vi "Warn.vi"(8 "NwarnIN":bool, 9 "HwarnIN":bool, 10 "warncontN":T1={"alarmliqN"=90.0, "warn?N"=FALSE, "lessthan?N"=FALSE}, 11 "warncontHe":T2={"alarmliqHe"=85.0, "warn?He"=FALSE, "lessthan?He"=FALSE}) -> (2 "warnNOUT":T1={"alarmliqN"=90.0, "warn?N"=FALSE, "lessthan?N"=FALSE}, 3 "warnHeOUT":T2={"alarmliqHe"=85.0, "warn?He"=FALSE, "lessthan?He"=FALSE})   [LabVIEW 2017, in "Level Meter.lvclass"]
uses:
  Level Meter.lvclass
  Global/Relative Sound Files.vi
panel:
  in  "turnoff":bool
  out "Nwarn":bool caption="LN"
  out "Hwarn":bool caption="LHe"
  in  "exit":bool
  out "disp":string
  out "warn2":bool
  out "warn1":bool
  # "Off"
  # "On"
  # "Greater"
  # "Less"
  # "Off"
  # "On"
  # "Greater"
  # "Less"
  # "Off"
  # "On"
  # "Greater"
  # "Less"
  # "Off"
  # "On"
  # "Greater"
  # "Less"
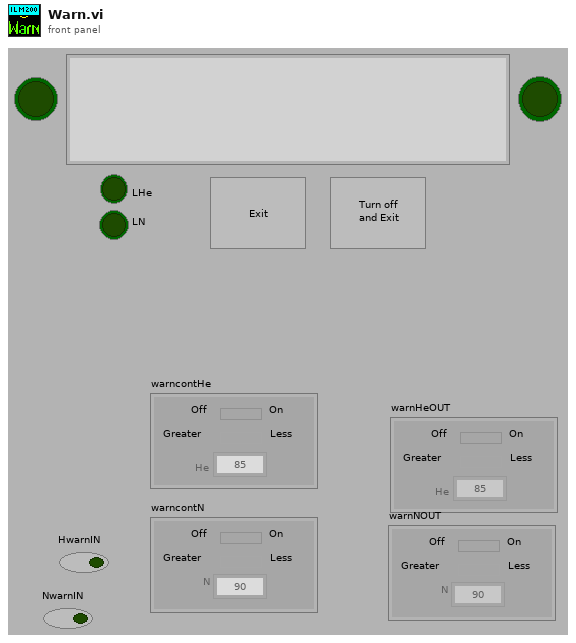
[diagram p1: front panel]
types:
  T1 = cluster{"alarmliqN":dbl, "warn?N":bool, "lessthan?N":bool}
  T2 = cluster{"alarmliqHe":dbl, "warn?He":bool, "lessthan?He":bool}
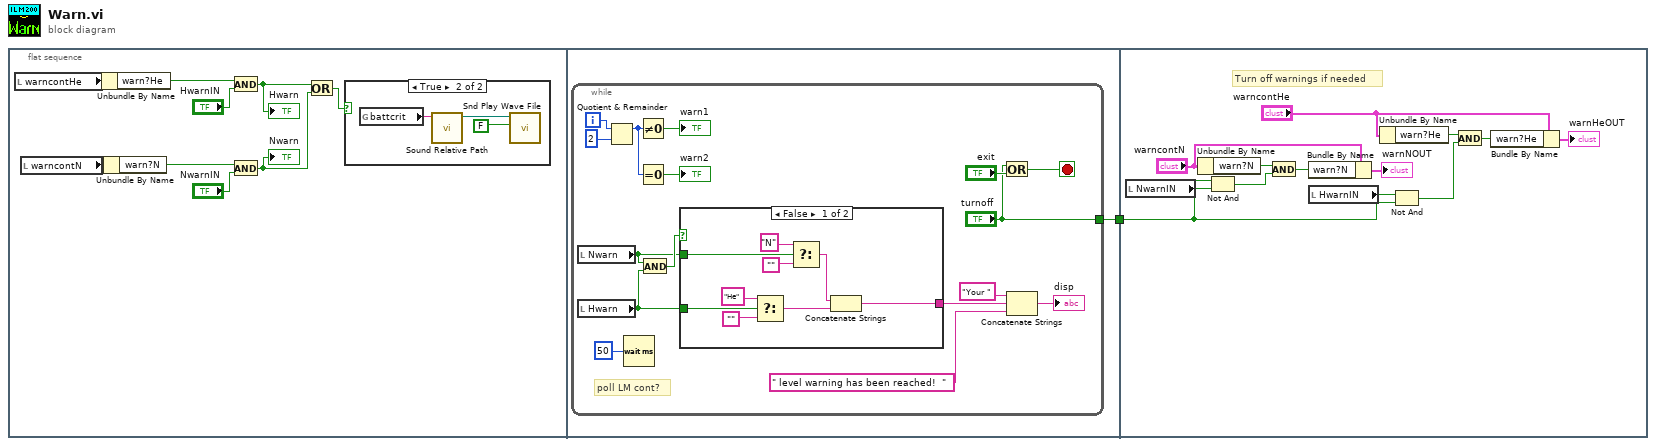
[diagram p0: block diagram]
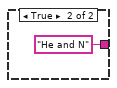
[diagram p3: hidden frame]
diagram:
  n1 = flat-sequence {
    tunnel: [w14] -> w1
    tunnel: w1 -> [w43]
    frame #0 {
      n2 = local read "warncontHe"() -> (w10:T2)
      n3 = local read "warncontN"() -> (w6:T1)
      n4 = Unbundle By Name(w10) -> ("warn?He"=w9:bool)
      n5 = Unbundle By Name(w6) -> ("warn?N"=w7:bool)
      n6 = And(x=w9, y="HwarnIN") -> (x .and. y?=w3:bool)
      "Hwarn" <- w3
      n7 = And(x=w7, y="NwarnIN") -> (x .and. y?=w2:bool)
      "Nwarn" <- w2
      n8 = Or(x=w3, y=w2) -> (x .or. y?=w4:bool)
      n9 = case shown="True" w4 {
        frame False {
        }
        frame True {
          n10 = global read "Relative Sound Files.vi" "battcrit"() -> (w12:string)
          n11 = call "Sound Relative Path.vi"("Sound"=w12) -> ("Relative Path"=w11:path)  [unwired: 10 in]
          n12 = call <vilib>:"Snd Play Wave File.vi"("wait until finish (T)"=FALSE, "wave file path"=w11) -> ()  [unwired: 1 in, 9 out]
        }
      }
    }
    frame #1 {
      n13 = while {
        tunnel: ["turnoff"] -> w14
        i -> [w30]
        stop <- w19 stop-if-true
        # "poll LM cont?"
        n14 = local read "Nwarn"() -> (w26:bool)
        n15 = local read "Hwarn"() -> (w25:bool)
        n16 = Quotient & Remainder(x=w30, y=2) -> (x-y*floor(x/y)=w17:i32)  [unwired: 1 out]
        n17 = Wait (ms)(milliseconds to wait=50) -> ()  [unwired: 1 out]
        n18 = Not Equal To 0?(x=w17) -> (x != 0?=→"warn1":bool)
        n19 = Equal To 0?(x=w17) -> (x = 0?=→"warn2":bool)
        n20 = And(x=w26, y=w25) -> (x .and. y?=w27:bool)
        n21 = case shown="False" w27 {
          tunnel: w26 -> [w39 _]
          tunnel: w25 -> [w38 _]
          tunnel: [w31 "He and N"] -> w24
          frame False {
            n22 = Select(t="He", s=w38, f="") -> (s? t:f=w37:string)
            n23 = Select(t="N", s=w39, f="") -> (s? t:f=w36:string)
            n24 = Concatenate Strings(w36, w37) -> (w31:string)
          }
          frame True {
          }
        }
        n25 = Or(x="turnoff", y="exit") -> (x .or. y?=w19:bool)
        n26 = Concatenate Strings("Your ", w24, " level warning has been reached!  ") -> (→"disp":string)
      }
    }
    frame #2 {
      # "Turn off warnings if needed"
      n27 = local read "NwarnIN"() -> (w44:bool)
      n28 = Unbundle By Name("warncontN") -> ("warn?N"=w46:bool)
      n29 = Not And(1:w44, 2:w43) -> (0:w42:bool)
      n30 = And(x=w46, y=w42) -> (x .and. y?=w45:bool)
      n31 = Bundle By Name(cluster="warncontN", "warn?N"=w45) -> (→"warnNOUT":T1)
      n32 = local read "HwarnIN"() -> (w41:bool)
      n33 = Unbundle By Name("warncontHe") -> ("warn?He"=w49:bool)
      n34 = Not And(1:w43, 2:w41) -> (0:w47:bool)
      n35 = And(x=w49, y=w47) -> (x .and. y?=w48:bool)
      n36 = Bundle By Name(cluster="warncontHe", "warn?He"=w48) -> (→"warnHeOUT":T2)
    }
  }
